vi "Display Text.vi"(8 "error in (no error)":errorcluster, 10 "Text":string, 11 "CLI in":refnum<class "CLI.lvclass">) -> (0 "error out":errorcluster, 3 "CLI out":refnum<class "CLI.lvclass">)   [LabVIEW 2020, in "neg-pkg-cli.lvlib" / "CLI.lvclass"]
uses:
  CLI.lvclass
  MGI Console/Source/Console/Console.lvclass
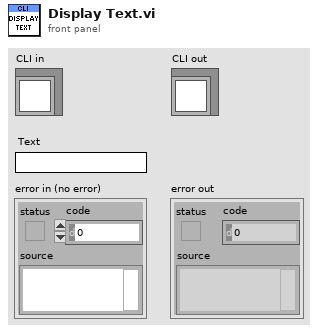
[diagram p1: front panel]
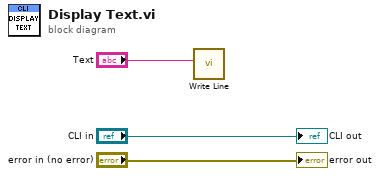
[diagram p0: block diagram]
diagram:
  n1 = call "Write Line.vi"("Line"="Text") -> ()  [unwired: 10 in, 1 out]
  "error out" <- "error in (no error)"
  "CLI out" <- "CLI in"
